vi "ExecEng_Report_AppendTextTableToReport.vi"(0 "report in":T3, 2 "measurement system":u16(ring) caption="measurement system\nfor column width (US)" items=["US", "Metric"], 3 "MS Office parameters":T2, 5 "column headers":string[](array[string]), 7 "row headers":string[](array[string]), 9 "text data":string[][](array[string]), 11 "error in (no error)":errorcluster, 12 "Column Width":sgl[](array[numeric]) format="%0.2f", 13 "separate page?":bool, 14 "show grid lines":bool=TRUE) -> (4 "report out":T3, 8 "range (wd) - start (xl)":T1, 10 "end (xl)":cluster{"row (xl) ":i32, "col (xl) ":i32}, 15 "error out":errorcluster)   [LabVIEW 2020]
doc: "Appends a 2D array to a report as a table with the given column width. You can use this polymorphic VI to append an array of strings or numbers. The data type you wire to the <B>text data</B> input determines the polymorphic instance to use."
uses:
  <vilib>/Utility/NIReport.llb/NI_ReportGenerationCore.lvlib
  <vilib>/addons/_office/NI_ReportGenerationToolkit.lvlib
  <vilib>/Utility/NIReport.llb/NI_report.lvclass
  <vilib>/Utility/NIReport.llb/Generate Report Object Reference.ctl
panel:
  in  "type specifier VI Refnum (for type only)":refnum<vi>
  in  "Excel_Insert_Table.vi":refnum<vi>
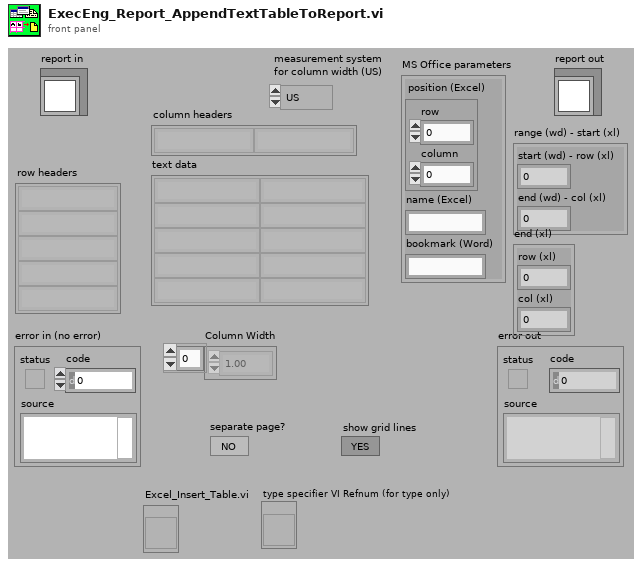
[diagram p1: front panel]
types:
  T1 = cluster{"start (wd) - row (xl) ":i32, "end (wd) - col (xl) ":i32}
  T2 = cluster{"position (Excel)":cluster{"row":i32, "column":i32}, "name (Excel) ":string, "bookmark (Word)":string}
  T3 = typedef "Generate Report Object Reference.ctl" = refnum<class "NI_report.lvclass">
  T4 = typedef "Generate Report Data Members.ctl" = cluster{"Title Text":string, "Header Text":string, "Body Text":string, "Footer Text":string, "Image List":path[], "NIReports.Report":refnum<k7>, "Report Type":enum16{"Standard Report", "HTML", "Word", "Excel"}, "Font Tag":string, "Word._Application":refnum<k7>, "Word._Document":refnum<k7>, "Word.Documents":refnum<k7>, "Word.InlineShapes":refnum<k7>, "Word.Tables":refnum<k7>, "Excel._Application":refnum<k7>, "Excel._Workbook":refnum<k7>, "Excel._Worksheet":refnum<k7>, "Excel.Sheets":refnum<k7>, "Excel.Shapes":refnum<k7>, "font":T5, "application directory":path, "application already open":bool, "from template?":bool}
  T5 = typedef "font.ctl" = cluster{"font name":string, "font size":dbl, "bold":u16, "italic":u16, "underline":u16, "strike through":u16, "font color":u32}
  T6 = typedef "Generate Report Object Reference.ctl" = refnum<k1>
  T7 = enum16{"Standard Report", "HTML", "Word", "Excel"}
  T8 = typedef "NISH Report.lvlib/Generate Report Object Reference.ctl" = refnum<k1>
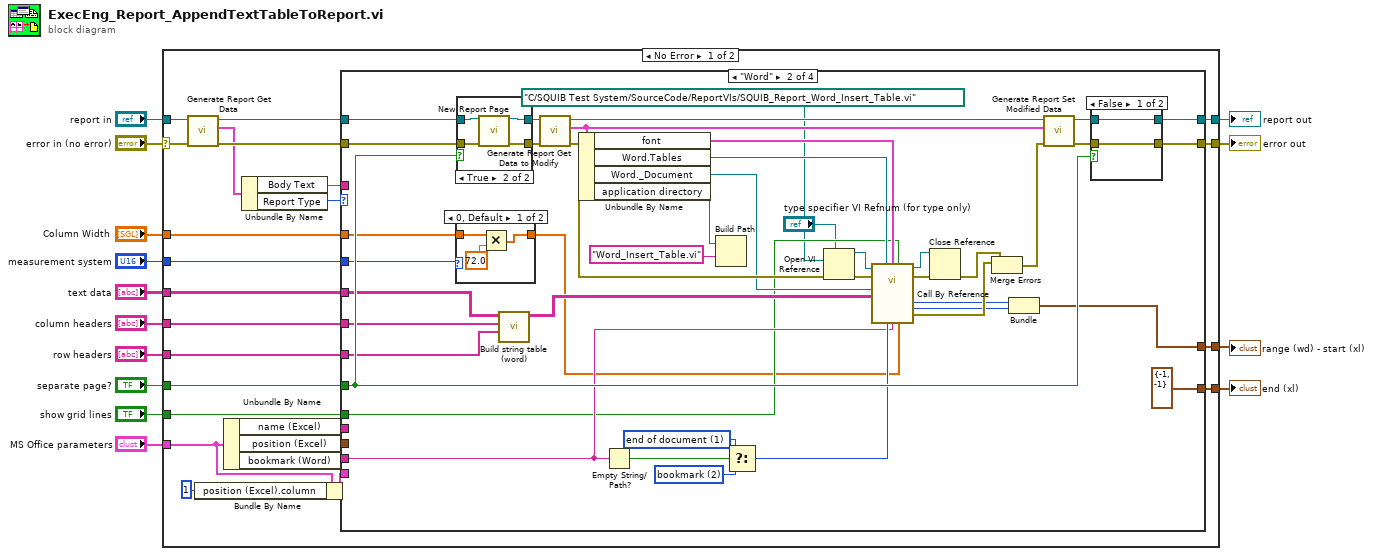
[diagram p0: block diagram]
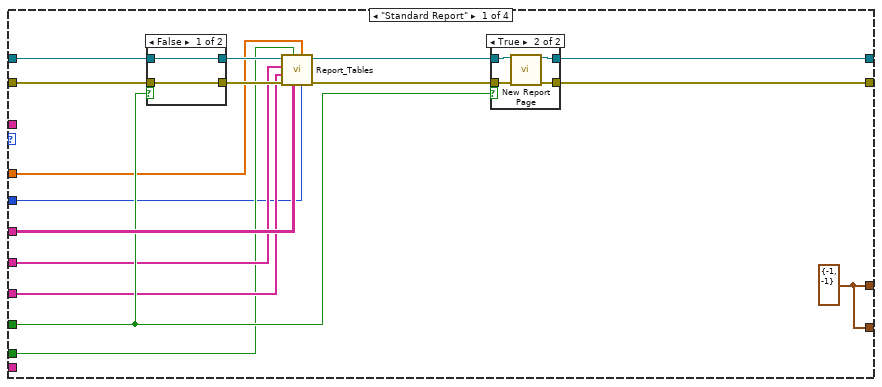
[diagram p2: hidden frame]
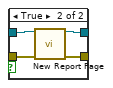
[diagram p4: hidden frame]
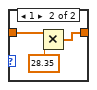
[diagram p5: hidden frame]
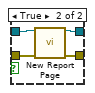
[diagram p6: hidden frame]
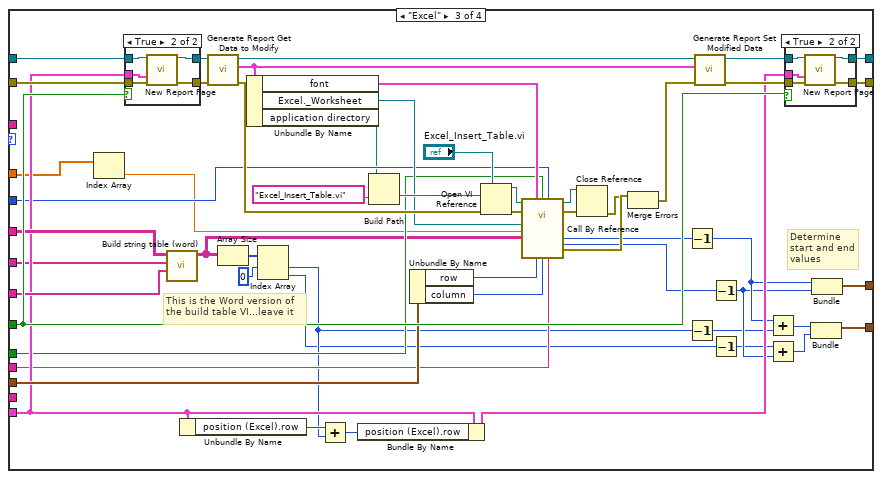
[diagram p8: hidden frame]
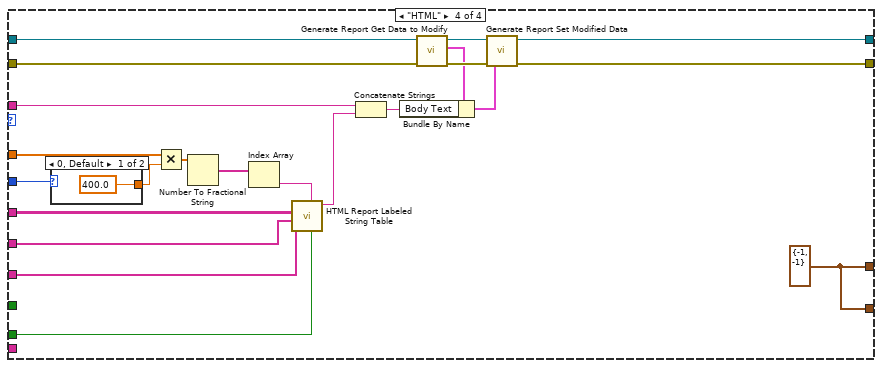
[diagram p11: hidden frame]
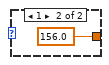
[diagram p12: hidden frame]
diagram:
  n1 = case shown="No Error" "error in (no error)" {
    selector: "error in (no error)" -> [w15 w221]
    tunnel: "text data" -> [w36 _]
    tunnel: "column headers" -> [w35 _]
    tunnel: "row headers" -> [w34 _]
    tunnel: "separate page?" -> [w32 _]
    tunnel: "Column Width" -> [w31 _]
    tunnel: "measurement system" -> [w30 _]
    tunnel: [w27 w221] -> w9
    tunnel: "report in" -> [w26 w222]
    tunnel: [w25 w222] -> w7
    tunnel: "show grid lines" -> [w24 _]
    tunnel: "MS Office parameters" -> [w19 _]
    tunnel: [w17 _] -> w4
    tunnel: [w16 _] -> w3
    frame No Error {
      n2 = call <vilib>:"Generate Report Get Data.vi"("error in (no error)"=w15, "report in"=w26) -> ("error out"=w38:errorcluster, "data"=w28:T4, "report out"=w29:T6)  [unwired: 2 in, 1 out]
      n3 = Bundle By Name(cluster=w19, "position (Excel).column"=1) -> (w21:T2)
      n4 = Unbundle By Name(w19) -> ("name (Excel)"=w18:string, "position (Excel)"=w22:cluster{"row":i32, "column":i32}, "bookmark (Word)"=w23:string)
      n5 = Unbundle By Name(w28) -> ("Body Text"=w33:string, "Report Type"=w37:T7)
      n6 = case shown="\"Word\"" w37 {
        tunnel: w38 -> [w43 w106 w181 w205]
        tunnel: [w48 w109 w136 w210] -> w27
        tunnel: w36 -> [w54 w97 w173 w218]
        tunnel: w35 -> [w49 w72 w131 w217]
        tunnel: w34 -> [w50 w96 w172 w216]
        tunnel: w33 -> [_ _ _ w215]
        tunnel: w32 -> [w51 w100 w175 _]
        tunnel: w31 -> [w41 w68 w129 w202]
        tunnel: w30 -> [w39 w98 w150 w201]
        tunnel: w29 -> [w44 w107 w182 w206]
        tunnel: [w47 w108 w135 w211] -> w25
        tunnel: w24 -> [w42 w82 w151 w200]
        tunnel: w23 -> [_ w85 _ _]
        tunnel: w22 -> [_ _ w171 _]
        tunnel: w21 -> [_ _ w170 _]
        tunnel: w18 -> [_ _ w154 _]
        tunnel: [w40 w78 w139 w199] -> w17
        tunnel: [w40 cluster{"row (xl)":i32, "col (xl)":i32} {"row (xl)"=-1, "col (xl)"=-1} ("end (xl)") w138 w199] -> w16
        frame "Standard Report" {
          w40 = cluster{"row (xl)":i32, "col (xl)":i32} {"row (xl)"=-1, "col (xl)"=-1} ("end (xl)")
          n7 = case shown="False" w51 {
            tunnel: w44 -> [w62 w66]
            tunnel: w43 -> [w61 w65]
            tunnel: [w62 w64] -> w53
            tunnel: [w61 w63] -> w52
            frame False {
            }
            frame True {
              n8 = call-dynamic "New Report Page.vi"("report in"=w66, "error in (no error)"=w65) -> ("report out"=w64:refnum<class "NI_report.lvclass">, "error out"=w63:errorcluster)  [unwired: 12 in]
            }
          }
          n9 = call "Report_Tables.vi"("Measurement System"=w39, "Column Width"=w41, "text data"=w54, "show grid lines"=w42, "error in (no error)"=w52, "row headers"=w50, "column headers"=w49, "report in"=w53) -> ("error out"=w46:errorcluster, "report out"=w45:T3)  [unwired: 2 in]
          n10 = case shown="True" w51 {
            tunnel: w45 -> [w56 w60]
            tunnel: w46 -> [w55 w59]
            tunnel: [w56 w58] -> w47
            tunnel: [w55 w57] -> w48
            frame False {
            }
            frame True {
              n11 = call-dynamic "New Report Page.vi"("report in"=w60, "error in (no error)"=w59) -> ("report out"=w58:T3, "error out"=w57:errorcluster)  [unwired: 12 in]
            }
          }
        }
        frame "Word" {
          w95 = u16 2 items=["begining of document", "end of document", "bookmark", "custom"] ("Insertion point")
          w94 = u16 1 items=["begining of document", "end of document", "bookmark", "custom"] ("Insertion point")
          n12 = case shown="0, Default" w98 {
            tunnel: w68 -> [w112 w114]
            tunnel: [w111 w113] -> w67
            frame 0, Default {
              n13 = Multiply(x=w112, y=sgl 72.0) -> (x*y=w111:sgl[])
            }
            frame 1 {
              n14 = Multiply(x=w114, y=28.35) -> (x*y=w113:dbl[])
            }
          }
          n15 = case shown="True" w100 {
            tunnel: w107 -> [w123 w127]
            tunnel: w106 -> [w122 w126]
            tunnel: [w123 w125] -> w104
            tunnel: [w122 w124] -> w105
            frame False {
            }
            frame True {
              n16 = call-dynamic "New Report Page.vi"("report in"=w127, "error in (no error)"=w126) -> ("report out"=w125:refnum<class "NI_report.lvclass">, "error out"=w124:errorcluster)  [unwired: 12 in]
            }
          }
          n17 = call <vilib>:"Build string table (word).vi"("row headers"=w96, "column headers"=w72, "text data"=w97) -> ("output table"=w87:string[][])  [unwired: 8 in]
          n18 = call <vilib>:"Generate Report Get Data to Modify.vi"("error in (no error)"=w105, "report in"=w104) -> ("error out"=w90:errorcluster, "data"=w99:T4, "report out"=w102:T6)  [unwired: 2 in, 1 out]
          n19 = Unbundle By Name(w99) -> ("font"=w83:T5, "Word.Tables"=w84:refnum<k7>, "Word._Document"=w89:refnum<k7>, "application directory"=w73:path)
          n20 = Empty String/Path?(string/path=w85) -> (empty?=w93:bool)
          n21 = Build Path(base path=w73, name or relative path="Word_Insert_Table.vi") -> ()  [unwired: 1 out]
          n22 = Select(t=w94, s=w93, f=w95) -> (s? t:f=w86:u16)
          n23 = Open VI Reference(type specifier VI Refnum (for type only)="type specifier VI Refnum (for type only)", vi path=path "C:/SQUIB Test System/SourceCode/ReportVIs/SQUIB_Report_Word_Insert_Table.vi" ("application directory"), error in (no error)=w90) -> (vi reference=w70:refnum<vi>, error out=w92:errorcluster)  [unwired: 3 in]
          n24 = call-by-ref "?"(reference=w70, error in=w92, "Document"=w89, "Tables"=w84, "font"=w83, "show grid lines"=w82, "Table data"=w87, "Insertion point"=w86, "Bookmark name"=w85, "ColumnWidthArray"=w67) -> (reference out=w74:refnum<vi>, error out=w76:errorcluster, "Start out"=w80:i32, "End out"=w79:i32, "error out"=w88:errorcluster)  [unwired: 5 in]
          n25 = Close Reference(reference=w74, error in (no error)=w76) -> (error out=w75:errorcluster)
          n26 = Merge Errors(w75, w88) -> (w81:errorcluster)
          n27 = Bundle("Start out"=w80, "End out"=w79) -> (w78:cluster{"Start out":i32, "End out":i32})  [unwired: 1 in]
          n28 = call "Generate Report Set Modified Data.vi"("error in (no error)"=w81, "data"=w99, "report in"=w102) -> ("error out"=w103:errorcluster, "report out"=w101:T8)  [unwired: 3 in]
          n29 = case shown="False" w100 {
            tunnel: [w117 w121] -> w108
            tunnel: [w116 w120] -> w109
            tunnel: w103 -> [w116 w119]
            tunnel: w101 -> [w117 w118]
            frame False {
            }
            frame True {
              n30 = call-dynamic "New Report Page.vi"("report in"=w118, "error in (no error)"=w119) -> ("report out"=w121:refnum<class "NI_report.lvclass">, "error out"=w120:errorcluster)  [unwired: 12 in]
            }
          }
        }
        frame "Excel" {
          # "This is the Word version of\nthe build table VI...leave it"
          # "Determine start and end values"
          n31 = Index Array(array=w129) -> (element=w128:sgl)  [unwired: 1 in]
          n32 = case shown="True" w175 {
            tunnel: w182 -> [w191 w196]
            tunnel: w181 -> [w190 w195]
            tunnel: [w191 w194] -> w179
            tunnel: [w190 w193] -> w180
            tunnel: w170 -> [_ w192]
            frame False {
            }
            frame True {
              n33 = call-dynamic "New Report Page.vi"("report in"=w196, "MS Office parameters"=w192, "error in (no error)"=w195) -> ("report out"=w194:refnum<class "NI_report.lvclass">, "error out"=w193:errorcluster)  [unwired: 11 in]
            }
          }
          n34 = call <vilib>:"Build string table (word).vi"("row headers"=w172, "column headers"=w131, "text data"=w173) -> ("output table"=w130:string[][])  [unwired: 8 in]
          n35 = Unbundle By Name(w170) -> ("position (Excel).row"=w169:i32)
          n36 = call <vilib>:"Generate Report Get Data to Modify.vi"("error in (no error)"=w180, "report in"=w179) -> ("error out"=w159:errorcluster, "data"=w174:T4, "report out"=w177:T6)  [unwired: 2 in, 1 out]
          n37 = Array Size(array=w130) -> (size(s)=w166:i32[])
          n38 = Unbundle By Name(w174) -> ("font"=w157:T5, "Excel._Worksheet"=w158:refnum<k7>, "application directory"=w137:path)
          n39 = Index Array(array=w166, index #1=0 ("Index")) -> (element #1=w141:i32, element #2=w140:i32)  [unwired: 1 in]
          n40 = Add(x=w169, y=w141) -> (x+y=w168:i32)
          n41 = Bundle By Name(cluster=w170, "position (Excel).row"=w168) -> (w167:T2)
          n42 = Build Path(base path=w137, name or relative path="Excel_Insert_Table.vi") -> (appended path=w161:path)
          n43 = Unbundle By Name(w171) -> ("row"=w156:i32, "column"=w155:i32)
          n44 = Open VI Reference(type specifier VI Refnum (for type only)="Excel_Insert_Table.vi", vi path=w161, error in (no error)=w159) -> (vi reference=w164:refnum<vi>, error out=w163:errorcluster)  [unwired: 3 in]
          n45 = call-by-ref "?"(reference=w164, error in=w163, "worksheet"=w158, "font"=w157, "show grid lines"=w151, "measurement system"=w150, "column width (1)"=w128, "table"=w130, "Start row"=w156, "Start column"=w155, "name"=w154) -> (reference out=w132:refnum<vi>, error out=w134:errorcluster, "Row"=w143:i32, "Column"=w142:i32, "error out"=w153:errorcluster)  [unwired: 4 in]
          n46 = Close Reference(reference=w132, error in (no error)=w134) -> (error out=w133:errorcluster)
          n47 = Merge Errors(w133, w153) -> (w152:errorcluster)
          n48 = Decrement(x=w143) -> (x-1=w147:i32)
          n49 = Decrement(x=w141) -> (x-1=w145:i32)
          n50 = call "Generate Report Set Modified Data.vi"("error in (no error)"=w152, "data"=w174, "report in"=w177) -> ("error out"=w178:errorcluster, "report out"=w176:T8)  [unwired: 3 in]
          n51 = Decrement(x=w142) -> (x-1=w146:i32)
          n52 = Decrement(x=w140) -> (x-1=w144:i32)
          n53 = Add(x=w147, y=w145) -> (x+y=w149:i32)
          n54 = Add(x=w144, y=w146) -> (x+y=w148:i32)
          n55 = case shown="True" w175 {
            tunnel: [w184 w189] -> w135
            tunnel: [w183 w188] -> w136
            tunnel: w178 -> [w183 w187]
            tunnel: w176 -> [w184 w186]
            tunnel: w167 -> [_ w185]
            frame False {
            }
            frame True {
              n56 = call-dynamic "New Report Page.vi"("report in"=w186, "MS Office parameters"=w185, "error in (no error)"=w187) -> ("report out"=w189:refnum<class "NI_report.lvclass">, "error out"=w188:errorcluster)  [unwired: 11 in]
            }
          }
          n57 = Bundle(w149, w148) -> (w138:cluster{i32, i32})  [unwired: 1 in]
          n58 = Bundle(w147, w146) -> (w139:cluster{i32, i32})  [unwired: 1 in]
        }
        frame "HTML" {
          w199 = cluster{"row (xl)":i32, "col (xl)":i32} {"row (xl)"=-1, "col (xl)"=-1} ("end (xl)")
          n59 = case shown="0, Default" w201 {
            tunnel: [400.0 ("y") 156.0 ("y")] -> w204
            frame 0, Default {
            }
            frame 1 {
            }
          }
          n60 = Multiply(x=w202, y=w204) -> (x*y=w203:dbl[])
          n61 = Number To Fractional String(number=w203) -> (F-format string=w198:string[])  [unwired: 3 in]
          n62 = Index Array(array=w198) -> (element=w197:string)  [unwired: 1 in]
          n63 = call <vilib>:"HTML Report Labeled String Table.vi"("Show Grid"=w200, "width"=w197, "row headers"=w216, "column headers"=w217, "table contents"=w218) -> ("HTML out"=w214:string)  [unwired: 6 in]
          n64 = Concatenate Strings(w215, w214) -> (w207:string)
          n65 = call <vilib>:"Generate Report Get Data to Modify.vi"("error in (no error)"=w205, "report in"=w206) -> ("error out"=w213:errorcluster, "data"=w209:T4, "report out"=w212:T6)  [unwired: 2 in, 1 out]
          n66 = Bundle By Name(cluster=w209, "Body Text"=w207) -> (w208:T4)
          n67 = call "Generate Report Set Modified Data.vi"("error in (no error)"=w213, "data"=w208, "report in"=w212) -> ("error out"=w210:errorcluster, "report out"=w211:T8)  [unwired: 3 in]
        }
      }
    }
    frame Error {
    }
  }
  "error out" <- w9
  "report out" <- w7
  "end (xl)" <- w3
  "range (wd) - start (xl)" <- w4
